vi "cDAQ Gas Pressure Convert AI Volt to Measurement.vi"(9 "Test Setup":T1, 11 "AI Voltage":T2) -> (3 "Mean measurement (in. H20)":dbl)   [LabVIEW 2014]
doc: "Converts AI voltage measurement to gas pressure reading"
uses:
  Type Definitions/cDAQ Instrument Sensor.ctl
panel:
  out "Std dev measurement":dbl
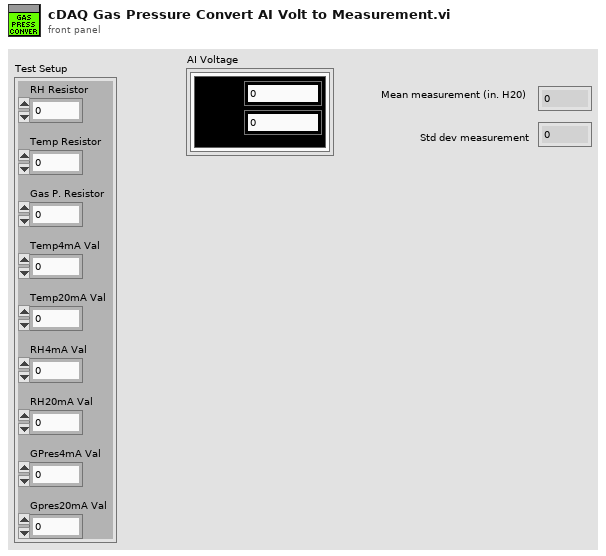
[diagram p1: front panel]
types:
  T1 = cluster{"RH Resistor":dbl, "Temp Resistor":dbl, "Gas P. Resistor":dbl, "Temp4mA Val":dbl, "Temp20mA Val":dbl, "RH4mA Val":dbl, "RH20mA Val":dbl, "GPres4mA Val":dbl, "Gpres20mA Val":dbl}
  T2 = typedef "cDAQ Instrument Sensor.ctl" = cluster{"Mean":dbl, " Std":dbl, "Color Box":u32}
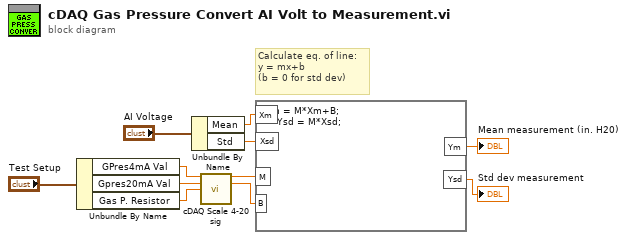
[diagram p0: block diagram]
diagram:
  # "Calculate eq. of line: \ny = mx+b \n(b = 0 for std dev)"
  n1 = Unbundle By Name("Test Setup") -> ("GPres4mA Val"=w3:dbl, "Gpres20mA Val"=w2:dbl, "Gas P. Resistor"=w1:dbl)
  n2 = Unbundle By Name("AI Voltage") -> ("Mean"=w8:dbl, "Std"=w6:dbl)
  n3 = call "cDAQ Scale 4-20 sig.vi"("4 mA y- value"=w3, "20 mA y-value"=w2, "Drop resistor"=w1) -> ("M"=w11:dbl, "B"=w10:dbl)  [unwired: 11 in]
  n4 = formula code="Ym = M*Xm+B;\n    Ysd = M*Xsd;"("M"=w11, "B"=w10, "Xm"=w8, "Xsd"=w6) -> ("Ym"=→"Mean measurement (in. H20)":dbl, "Ysd"=→"Std dev measurement":dbl)
